vi "BPSK_rxCRC.vi"(8 "error in (no error)":errorcluster caption="错误输入（无错误）", 10 "input_data":dbl[](array[numeric]) format="%#_13g", 11 "PathIn":path) -> (0 "error out":errorcluster caption="错误输出", 1 "CRC_flag":i32, 2 "out_data":dbl[](array[numeric]), 3 "PathOut":path)   [LabVIEW 2015]
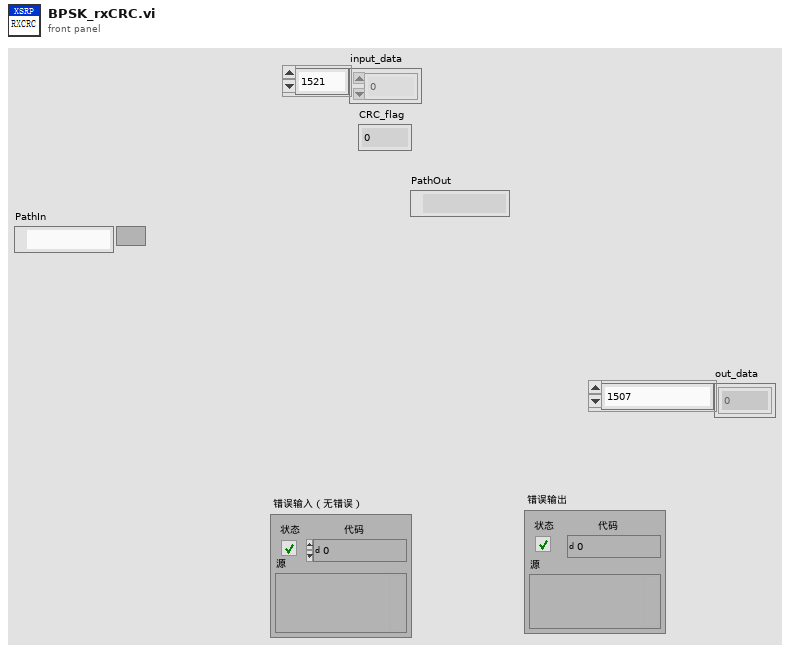
[diagram p1: front panel]
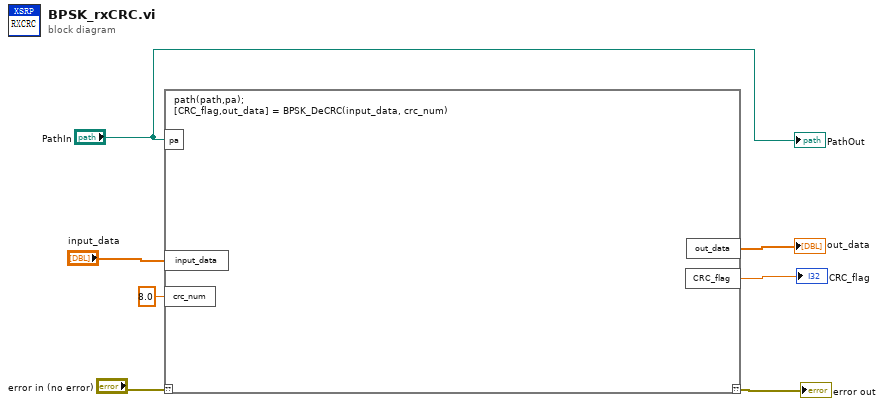
[diagram p0: block diagram]
diagram:
  n1 = script code="path(path,pa);\n[CRC_flag,out_data] = BPSK_DeCRC(input_data, crc_num)"("??"="error in (no error)", "pa"="PathIn", "input_data"="input_data", "crc_num"=8.0 ("Real")) -> ("??"=→"error out":errorcluster, "out_data"=→"out_data":dbl[], "CRC_flag"=→"CRC_flag":dbl)
  "PathOut" <- "PathIn"
